vi "Unrecognized CLI Command--error.vi"() -> (0 "error out":errorcluster)   [LabVIEW 2025]
doc: "Indicates that the specified CLI command does not exist."
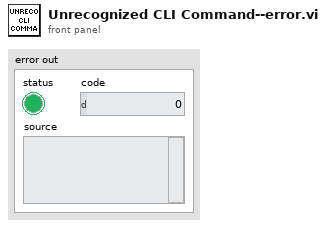
[diagram p1: front panel]
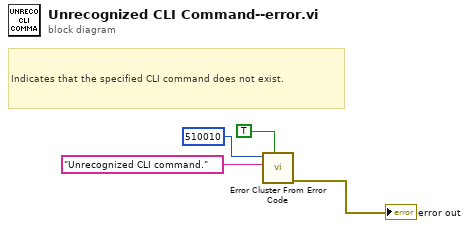
[diagram p0: block diagram]
diagram:
  # "Indicates that the specified CLI command does not exist."
  n1 = call <vilib>:"Error Cluster From Error Code.vi"("show call chain? (False)"=TRUE, "error message (\"\")"="Unrecognized CLI command." ("error message (\"\")"), "error code (0)"=510010) -> ("error out"=→"error out":errorcluster)  [unwired: 6 in]
